vi "Add CSVs to Test List.vi"(8 "error in (no error)":errorcluster, 9 "Array":path[](array[path]), 10 "TopLevel in in":T1, 11 "QSM in in":string[](array[string])) -> (0 "error out":errorcluster, 2 "TopLevel in out":T1, 3 "QSM in out":string[](array[string]))   [LabVIEW 2011]
uses:
  Controls/Top Level Control.ctl
  <vilib>/NI/AMC/Message Queue.ctl
  <vilib>/NI/AMC/Message.ctl
  <vilib>/NI/Tools/Keyed Array/KeyedArray.ctl
  Controls/ListBox Test Record.ctl
  Controls/DVR of CSV Tests Data.ctl
  Controls/CSVs Tests Data.ctl
  Controls/Test Column Data.ctl
  Controls/Options DVR.ctl
  Controls/Options.ctl
  <userlib>/_OpenG.lib/array/array.llb/Conditional Auto-Indexing Tunnel (String)__ogtk.vi
  <userlib>/_OpenG.lib/array/array.llb/Conditional Auto-Indexing Tunnel (Path)__ogtk.vi
  <vilib>/NI/Tools/Keyed Array/Tools_KeyedArray.lvlib
  <vilib>/NI/AMC/AMC.lvlib
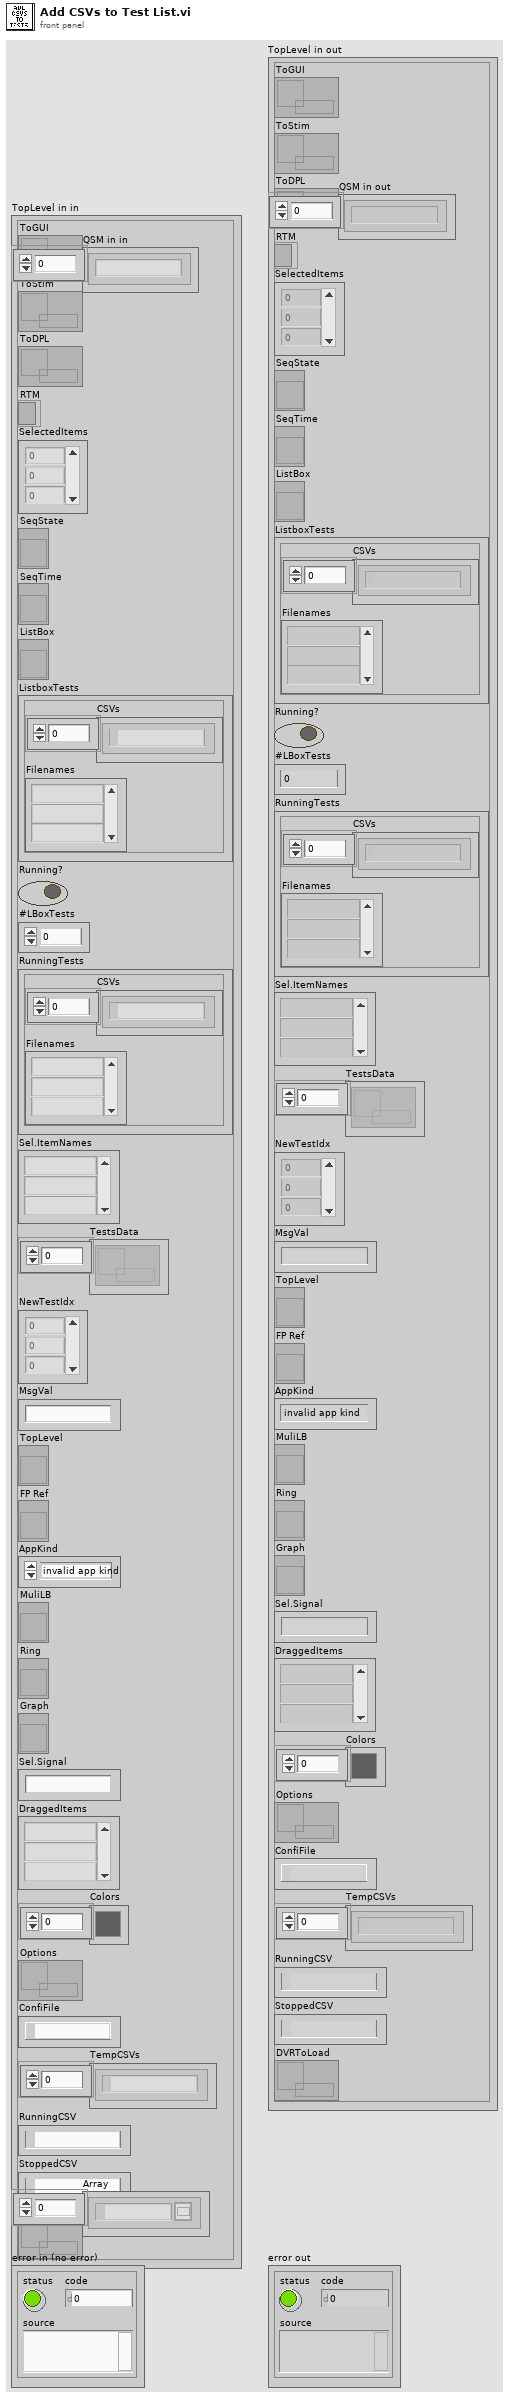
[diagram p1: front panel]
types:
  T1 = typedef "Top Level Control.ctl" = cluster{"ToGUI":T2, "ToStim":T2, "ToDPL":T2, "RTM":refnum<k9>, "SelectedItems":i32[], "SeqState":refnum<vi>, "SeqTime":refnum<vi>, "ListBox":refnum<vi>, "ListboxTests":T3, "Running?":bool, "#LBoxTests":i32, "RunningTests":T3, "Sel.ItemNames":string[], "TestsData":T4[], "NewTestIdx":i32[], "MsgVal":string, "TopLevel":refnum<vi>, "FP Ref":refnum<vi>, "AppKind":enum32{"invalid app kind", "Development System", "Run Time System", "Student Edition", "Embedded LabVIEW", "Evaluation", "Custom"}, "MuliLB":refnum<vi>, "Ring":refnum<vi>, "Graph":refnum<vi>, "Sel.Signal":string, "DraggedItems":string[], "Colors":u32[], "Options":T5, "ConfiFile":path, "TempCSVs":path[], "RunningCSV":path, "StoppedCSV":path, "DVRToLoad":T4}
  T2 = typedef "AMC.lvlib/Message Queue.ctl" = refnum<queue>
  T3 = typedef "ListBox Test Record.ctl" = cluster{"CSVs":path[], "Filenames":string[]}
  T4 = typedef "DVR of CSV Tests Data.ctl" = refnum<data-value>
  T5 = typedef "Options DVR.ctl" = refnum<data-value>
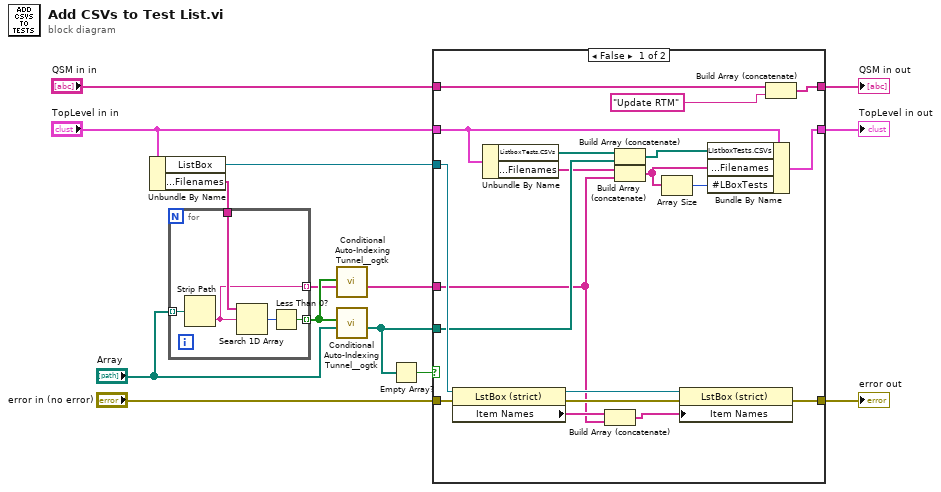
[diagram p0: block diagram]
diagram:
  n1 = Unbundle By Name("TopLevel in in") -> ("ListBox"=w1:refnum<vi>, "ListboxTests.Filenames"=w2:string[])
  n2 = for {
    tunnel: "Array" -> [w19] mode=indexing
    tunnel: w2 -> [w17]
    tunnel: [w16] -> w5 mode=indexing
    tunnel: [w15] -> w4 mode=indexing
    n3 = Strip Path(path=w19) -> (name=w15:string)  [unwired: 1 out]
    n4 = Search 1D Array(1D array=w17, element=w15) -> (index of element=w18:i32)  [unwired: 1 in]
    n5 = Less Than 0?(x=w18) -> (x < 0?=w16:bool)
  }
  n6 = call-poly <userlib>:"Conditional Auto-Indexing Tunnel__ogtk.vi"("Array in"=w4, "Elements to keep"=w5) -> ("Filtered Array out"=w3:string[])  [unwired: 5 in]
  n7 = call-poly <userlib>:"Conditional Auto-Indexing Tunnel__ogtk.vi"("Array in"="Array", "Elements to keep"=w5) -> ("Filtered Array out"=w6:path[])  [unwired: 5 in]
  n8 = Empty Array?(array=w6) -> (empty?=w7:bool)
  n9 = case shown="False" w7 {
    tunnel: "error in (no error)" -> [w38 w41]
    tunnel: [w33 w41] -> w10
    tunnel: w6 -> [w26 _]
    tunnel: [w31 w40] -> w11
    tunnel: "QSM in in" -> [w32 w40]
    tunnel: w1 -> [w29 _]
    tunnel: [w22 w39] -> w13
    tunnel: "TopLevel in in" -> [w28 w39]
    tunnel: w3 -> [w24 _]
    frame False {
      n10 = property on="Property Node" class="LstBox (strict)"(reference=w29, error in=w38) -> (reference out=w34:refnum<vi>, error out=w35:errorcluster, "Item Names"=w37:string[])
      n11 = Unbundle By Name(w28) -> ("ListboxTests.CSVs"=w27:path[], "ListboxTests.Filenames"=w25:string[])
      n12 = Build Array (concatenate)(w37, w24) -> (w36:string[])
      n13 = Build Array (concatenate)(w27, w26) -> (w23:path[])
      n14 = Build Array (concatenate)(w25, w24) -> (w21:string[])
      n15 = Array Size(array=w21) -> (size(s)=w20:i32)
      n16 = property on="Property Node" class="LstBox (strict)"(reference=w34, error in=w35, "Item Names"=w36) -> (error out=w33:errorcluster)  [unwired: 1 out]
      n17 = Bundle By Name(cluster=w28, "ListboxTests.CSVs"=w23, "ListboxTests.Filenames"=w21, "#LBoxTests"=w20) -> (w22:T1)
      n18 = Build Array (concatenate)(w32, "Update RTM" ("button label")) -> (w31:string[])
    }
    frame True {
    }
  }
  "TopLevel in out" <- w13
  "QSM in out" <- w11
  "error out" <- w10
